vi "noise.vi"() -> ()   [LabVIEW 2009]
panel:
  in  "Q":dbl
  out "所望波":cluster{dbl[], dbl[]}(graph)
  out "スペクトルアナライザ":cluster{dbl[], dbl[]}(graph)
  out "送信波":cluster{dbl[], dbl[]}(graph)
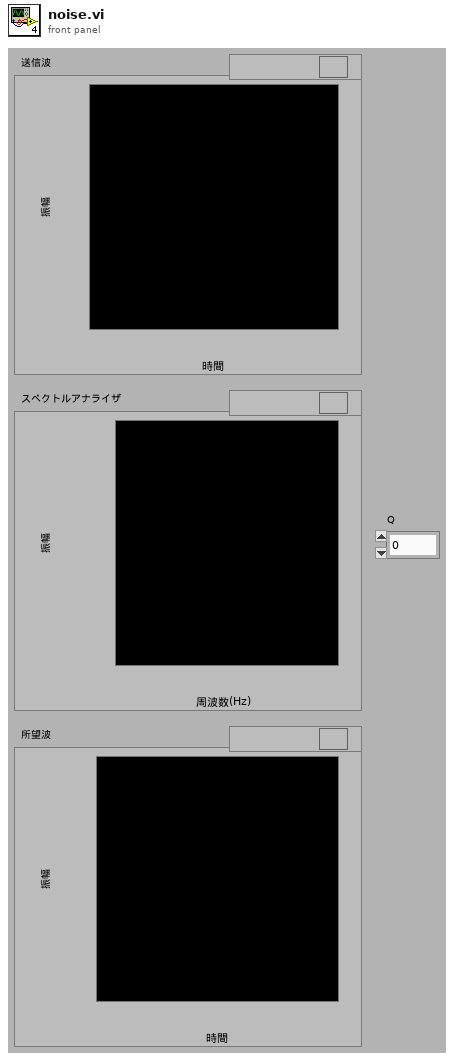
[diagram p1: front panel]
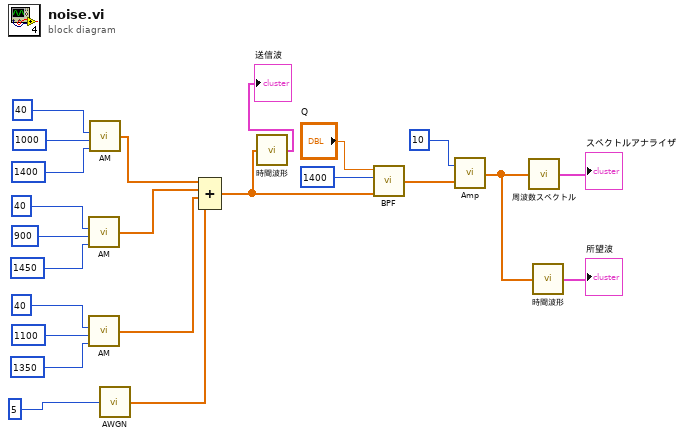
[diagram p0: block diagram]
diagram:
  n1 = call "AM.vi"("変調度 [%]"=40, "変調周波数 [Hz]"=900, "搬送波周波数 [kHz]"=1450) -> ("変調波"=w13:dbl[])  [unwired: 2 in]
  n2 = call "AM.vi"("変調度 [%]"=40, "変調周波数 [Hz]"=1100, "搬送波周波数 [kHz]"=1350) -> ("変調波"=w12:dbl[])  [unwired: 2 in]
  n3 = call "AM.vi"("変調度 [%]"=40, "変調周波数 [Hz]"=1000, "搬送波周波数 [kHz]"=1400) -> ("変調波"=w14:dbl[])  [unwired: 2 in]
  n4 = call "AWGN.vi"("振幅値"=5) -> ("出力"=w11:dbl[])
  n5 = Compound Arithmetic op=ADD(w14, w13, w12, w11) -> (w8:dbl[])
  n6 = call "時間波形.vi"("入力"=w8) -> ("時間波形"=→"送信波":cluster{dbl[], dbl[]})
  n7 = call "BPF.vi"("X"=w8, "中心周波数 [kHz]"=1400, "Q"="Q") -> ("BPF出力"=w6:dbl[])  [unwired: 1 in]
  n8 = call "Amp.vi"("入力"=w6, "増幅率"=10) -> ("出力"=w3:dbl[])
  n9 = call "周波数スペクトル.vi"("入力"=w3) -> ("周波数スペクトル"=→"スペクトルアナライザ":cluster{dbl[], dbl[]})
  n10 = call "時間波形.vi"("入力"=w3) -> ("時間波形"=→"所望波":cluster{dbl[], dbl[]})
